vi "Read Alarm Status.vi"(8 "error in":errorcluster, 11 "Value in":refnum<class "Value.lvclass">) -> (0 "error out":errorcluster, 1 "has alarm status?":bool, 2 "alarm status":T1, 3 "Value out":refnum<class "Value.lvclass">)   [LabVIEW 2020, in "Value.lvlib" / "Value.lvclass"]
uses:
  Value.lvclass
  Value.lvclass/Value.ctl
  <vilib>/addons/Tools/Unicode/UTF8 Tools.lvlib
  Alarm Status.ctl
  Value.lvlib
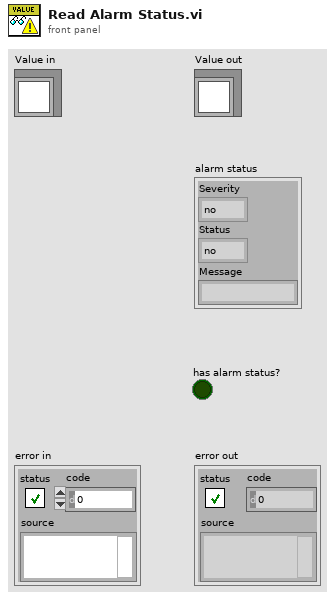
[diagram p1: front panel]
types:
  T1 = typedef "Value.lvlib/Alarm Status.ctl" = cluster{"Severity":enum32{"no", "minor", "major", "record", "invalid", "undefined", ""}, "Status":enum32{"no", "device", "driver", "record", "db", "conf", "undefined", "client"}, "Message":string}
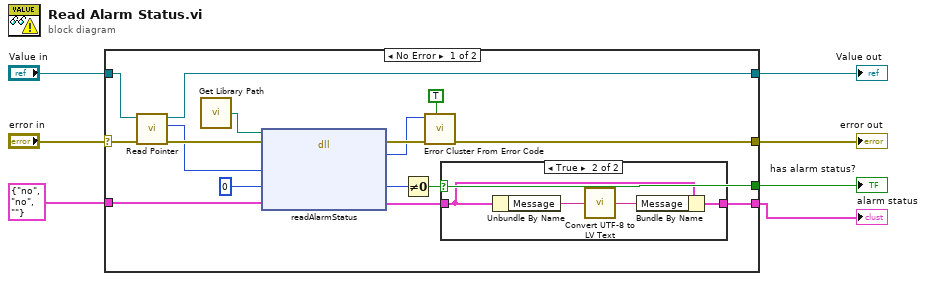
[diagram p0: block diagram]
diagram:
  n1 = case shown="No Error" "error in" {
    selector: "error in" -> [w18 w30]
    tunnel: [w19 w30] -> w7
    tunnel: "Value in" -> [w16 w29]
    tunnel: [w14 w29] -> w4
    tunnel: T1 {"Severity"=enum."no", "Status"=enum."no", "Message"=""} ("Alarm") -> [w13 _]
    tunnel: [w10 _] -> w3
    tunnel: [w8 _] -> w1
    frame No Error {
      n2 = call-dynamic "Read Pointer.vi"("error in (no error)"=w18, "Value in"=w16) -> ("error out"=w17:errorcluster, "pointer"=w15:i64, "Value out"=w14:refnum<class "Value.lvclass">)  [unwired: 7 in]
      n3 = call "Get Library Path.vi"() -> ("Path"=w23:path)  [unwired: 1 in]
      n4 = dll-call lib="?" fn="readAlarmStatus"(path in=w23, error in=w17, "value"=w15, "has alarm status?"=i16 0 ("has display metadata?"), "alarm status"=w13) -> (error out=w21:errorcluster, "err_code"=w20:i32, "has alarm status?"=w12:i16, "alarm status"=w9:T1)  [unwired: 2 in, 1 out]
      n5 = Not Equal To 0?(x=w12) -> (x != 0?=w10:bool)
      n6 = call <vilib>:"Error Cluster From Error Code.vi"("show call chain? (False)"=TRUE, "error in (no error)"=w21, "error code (0)"=w20) -> ("error out"=w19:errorcluster)  [unwired: 6 in]
      n7 = case shown="True" w10 {
        tunnel: w9 -> [w24 w27]
        tunnel: [w24 w25] -> w8
        frame False {
        }
        frame True {
          n8 = Unbundle By Name(w27) -> ("Message"=w28:string)
          n9 = call <vilib>:"Convert UTF-8 to LV Text.vi"("UTF-8 Text"=w28) -> ("LV Text"=w26:string)  [unwired: 13 in, 1 out]
          n10 = Bundle By Name(cluster=w27, "Message"=w26) -> (w25:T1)
        }
      }
    }
    frame Error {
    }
  }
  "error out" <- w7
  "Value out" <- w4
  "has alarm status?" <- w3
  "alarm status" <- w1
